vi "Actor Core.vi"(8 "error in":errorcluster, 11 "UIA_ChildTest in":refnum<class "UIA_ChildTest.lvclass">) -> (0 "error out":errorcluster, 3 "Actor out":refnum<class "Actor.lvclass">)   [LabVIEW 2020, in "UIA_ChildTest.lvlib" / "UIA_ChildTest.lvclass"]
doc: "(<B>Filename</B>: Actor Framework.lvlib:Actor.lvclass:Actor Core.vi)\n\nReceives messages to the actor, reacts to them, and initiates any error handling that may shut the actor down.\n\nDescendant classes may override this VI to append parallel tasks for the actor to complete while it handles messages. Overrides use the Call Parent Method node."
uses:
  UIA_ChildTest.lvclass
  D:/Projets/STEP AT/UI Actor/UI_Actor/UI_Actor/UI_Actor.lvclass
  support/Actor Framework.lvlibp/1abvi3w/vi.lib/ActorFramework/Actor/Actor.lvclass
  UI_Actor/UI_Actor/UI_Actor.lvclass/UI_Actor.ctl
  UI_Actor/UI_Actor/Read AppVersion.vi
  UI_Actor/UI_Actor/UI_Actor.lvclass
panel:
  out "S2.indic":dbl caption="B2 indic"
  out "AppVersion":string
  out "S2.Time":timestamp
  in  "S1.Enum":enum16{""}(ring)
  in  "S1.Ring":u16(ring)
  out "S1.Indic2":bool caption="Indic2"
  out "S1.Indic1":dbl caption="Indic1"
  in  "S1.Ctl2":dbl caption="Ctl2"
  in  "S1.Ctl1":dbl caption="Ctl1"
  in  "Cluster":cluster{"S1.Clust num":dbl}
  out "S1.Slide":u8(slide) caption="Slide" scale=0.0..100.0
  in  "Tab Control":enum32{"Page 1", "Page 2"}(tab)
  out "S1.Indic3 in tab ctl":dbl caption="Indic3 in tab ctl"
  # "UI ACTOR CHILDTEST\n\nINTERFACE DE TEST"
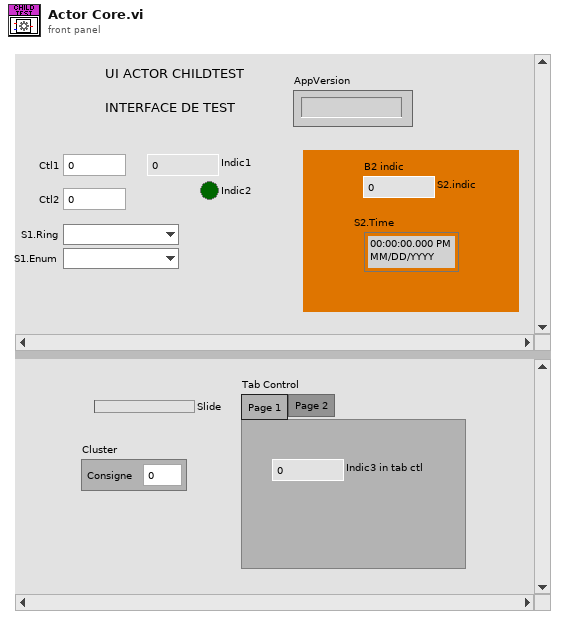
[diagram p1: front panel]
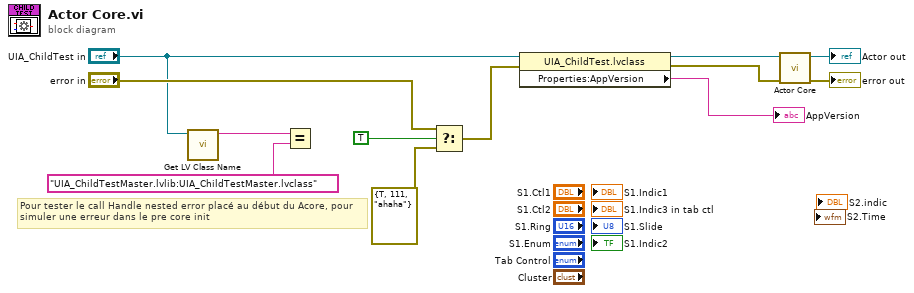
[diagram p0: block diagram]
diagram:
  # "Pour tester le call Handle nested error placé au début du Acore, pour simuler une erreur dans le pre core init"
  n1 = call <vilib>:"Get LV Class Name.vi"("object"="UIA_ChildTest in") -> ("class name"=w3:string)  [unwired: 9 in, 1 out]
  n2 = Equal?(x=w3, y="UIA_ChildTestMaster.lvlib:UIA_ChildTestMaster.lvclass") -> ()  [unwired: 1 out]
  n3 = Select(t="error in", s=TRUE, f=errorcluster {"status"=TRUE, "code"=111, "source"="ahaha"} ("error in")) -> (s? t:f=w5:errorcluster)
  n4 = property class="UIA_ChildTest.lvclass"(reference="UIA_ChildTest in", error in=w5) -> (reference out=w10:refnum<class "UIA_ChildTest.lvclass">, error out=w8:errorcluster, "Properties:AppVersion"=→"AppVersion":string)
  n5 = call-parent "Actor Core.vi"("error in"=w8, "UI_Actor in"=w10) -> ("error out"=→"error out":errorcluster, "Actor out"=→"Actor out":refnum<class "Actor.lvclass">)  [unwired: 8 in]
